vi "SSL Vision Log Player.vi"() -> ()   [LabVIEW 2016]
uses:
  SSL Referee Game Status.ctl
  GUI/IA Robot Line Display.ctl
  Filters/Estimadores.ctl
  SSL/SSL Field State.ctl
  SSL Detection Frame.ctl
  SSL Detection Robot.ctl
  SSL Detection Ball.ctl
  <extravilib>/ChannelInstances/Lossy Stream-t'SSL Field State.ctl'/Write With Abort.vi
  <extravilib>/ChannelInstances/Lossy Stream-t'SSL Referee Game Status.ctl'/Write With Abort.vi
  <extravilib>/ChannelInstances/Lossy Stream-t'SSL Referee Game Status.ctl'/Read With Abort.vi
  <extravilib>/ChannelInstances/Lossy Stream-t'SSL Field State.ctl'/Read With Abort.vi
  <extravilib>/ChannelInstances/Lossy Stream-t'AI Input.ctl'/Write With Abort.vi
  <extravilib>/ChannelInstances/Lossy Stream-t'AI Input.ctl'/Read With Abort.vi
  <extravilib>/ChannelInstances/Lossy Stream-t'SSL Field State.ctl'/Endpoint.vi
  <extravilib>/ChannelInstances/Lossy Stream-t'SSL Referee Game Status.ctl'/Endpoint.vi
  <extravilib>/ChannelInstances/Lossy Stream-t'AI Input.ctl'/Endpoint.vi
  <extravilib>/ChannelInstances/Lossy Stream-t'AI Input.ctl'/Instantiate.vi
  <extravilib>/ChannelInstances/Lossy Stream-t'AI Input.ctl'/)Channel.vi
  <resource>/ChannelSupport/_ChannelSupport/WaitIfNeeded.vi
  <extravilib>/ChannelInstances/Lossy Stream-t'SSL Referee Game Status.ctl'/Instantiate.vi
  <extravilib>/ChannelInstances/Lossy Stream-t'SSL Field State.ctl'/Instantiate.vi
  <extravilib>/ChannelInstances/Lossy Stream-t'SSL Referee Game Status.ctl'/)Channel.vi
  <extravilib>/ChannelInstances/Lossy Stream-t'SSL Field State.ctl'/)Channel.vi
  <extravilib>/ChannelInstances/Lossy Stream-a[.](u8)/Instantiate.vi
  <extravilib>/ChannelInstances/Stream-a[.](u8)/Instantiate.vi
  <extravilib>/ChannelInstances/Lossy Stream-t'SSL Referee Game Status.ctl'.lvlib
  <extravilib>/ChannelInstances/Lossy Stream-t'AI Input.ctl'.lvlib
  <extravilib>/ChannelInstances/Lossy Stream-t'SSL Field State.ctl'.lvlib
panel:
  in  "Estimador":T1
  out "Time Stamp":timestamp format="%<%.3X %x>T"
  out "error out 5":errorcluster
  out "error out 4":errorcluster
  out "Boolean":bool
  out "error out 3":errorcluster
  in  "Boolean 4":bool
  out "Boolean 3":bool
  in  "Port:":u16=10001
  in  "SSL Referee Address:":string="224.5.92.5"
  in  "Slide":i64(slide) min=0 max=47299339 scale=0.0..47299339.0
  out "offset (in bytes)":i64 format="%.3p"
  out "size (in bytes)":i64 format="%.3p"
  out "Boolean 2":bool
  in  "Modo":bool
  in  "Port:":u16=10020
  in  "file path (use dialog)":path=path "E:/Media/2016-07-01_cmdragons_immortals.log"
  in  "SSL Vision Address:":string="224.5.23.2"
  out "Role Playing FPS":dbl
  out "Total Delay":dbl format="%#.5g"
  in  "Goalie":string(combo)="Auto"
  in  "Command":string(combo)="Auto"
  in  "Time":enum16{"Azul", "Amarelo"}(ring) caption="Enum"
  in  "Lado":enum16{"Esquerdo", "Direito"}(ring) caption="Enum"
  in  "Role Decisor":enum16{"Simple Role Decisor", "No Role Decisor"}(ring)
  out "Game Status":T2={"Stage"="Normal First Half Pre", "Command"="Stop", "Time Left"=0.0, "Yellow Team"="", "Blue Team"="", "Yellow Score"=0, "Blue Score"=0, "Yellow Red Cards"=0, "Blue Red Cards"=0, "Yellow Yellow Cards"=0, "Blue Yellow Cards"=0, "Yellow Timeouts Left"=0, "Blue Timeouts Left"=0, "Yellow Timeout Remaining"=0.0, "Blue Timeout Remaining"=0.0, "Yellow Goalie Id"=0, "Blue Goalie Id"=0, "Time"=timestamp(2082758400 s since 1904-01-01)} {"Time" format="%<%.3X %x>T"; "Blue Timeout Remaining" format="%<%M:%S>t"; "Yellow Timeout Remaining" format="%<%M:%S>t"; "Time Left" format="%<%M:%S>t"}
  out "error out":errorcluster
  in  "Tab Control":enum32{"Robots", "Transmissão"}(tab)
  out "GUI Robot Array":T3[](array[typedef])
  in  "Serial TX":bool
  in  "UDP TX":bool=TRUE
  in  "Address:":string="127.0.0.1"
  in  "Port:":u16=20011
  in  "Porta:":refnum<visa-resource-name>
  out "Comm FPS":dbl
  out "error out 2":errorcluster
  # "UDP"
  # "LOG"
  # "Score"
  # "Red Cards"
  # "Yellow Cards"
  # "Timeouts Left"
  # "Timeout Remaining"
  # "Goalie ID"
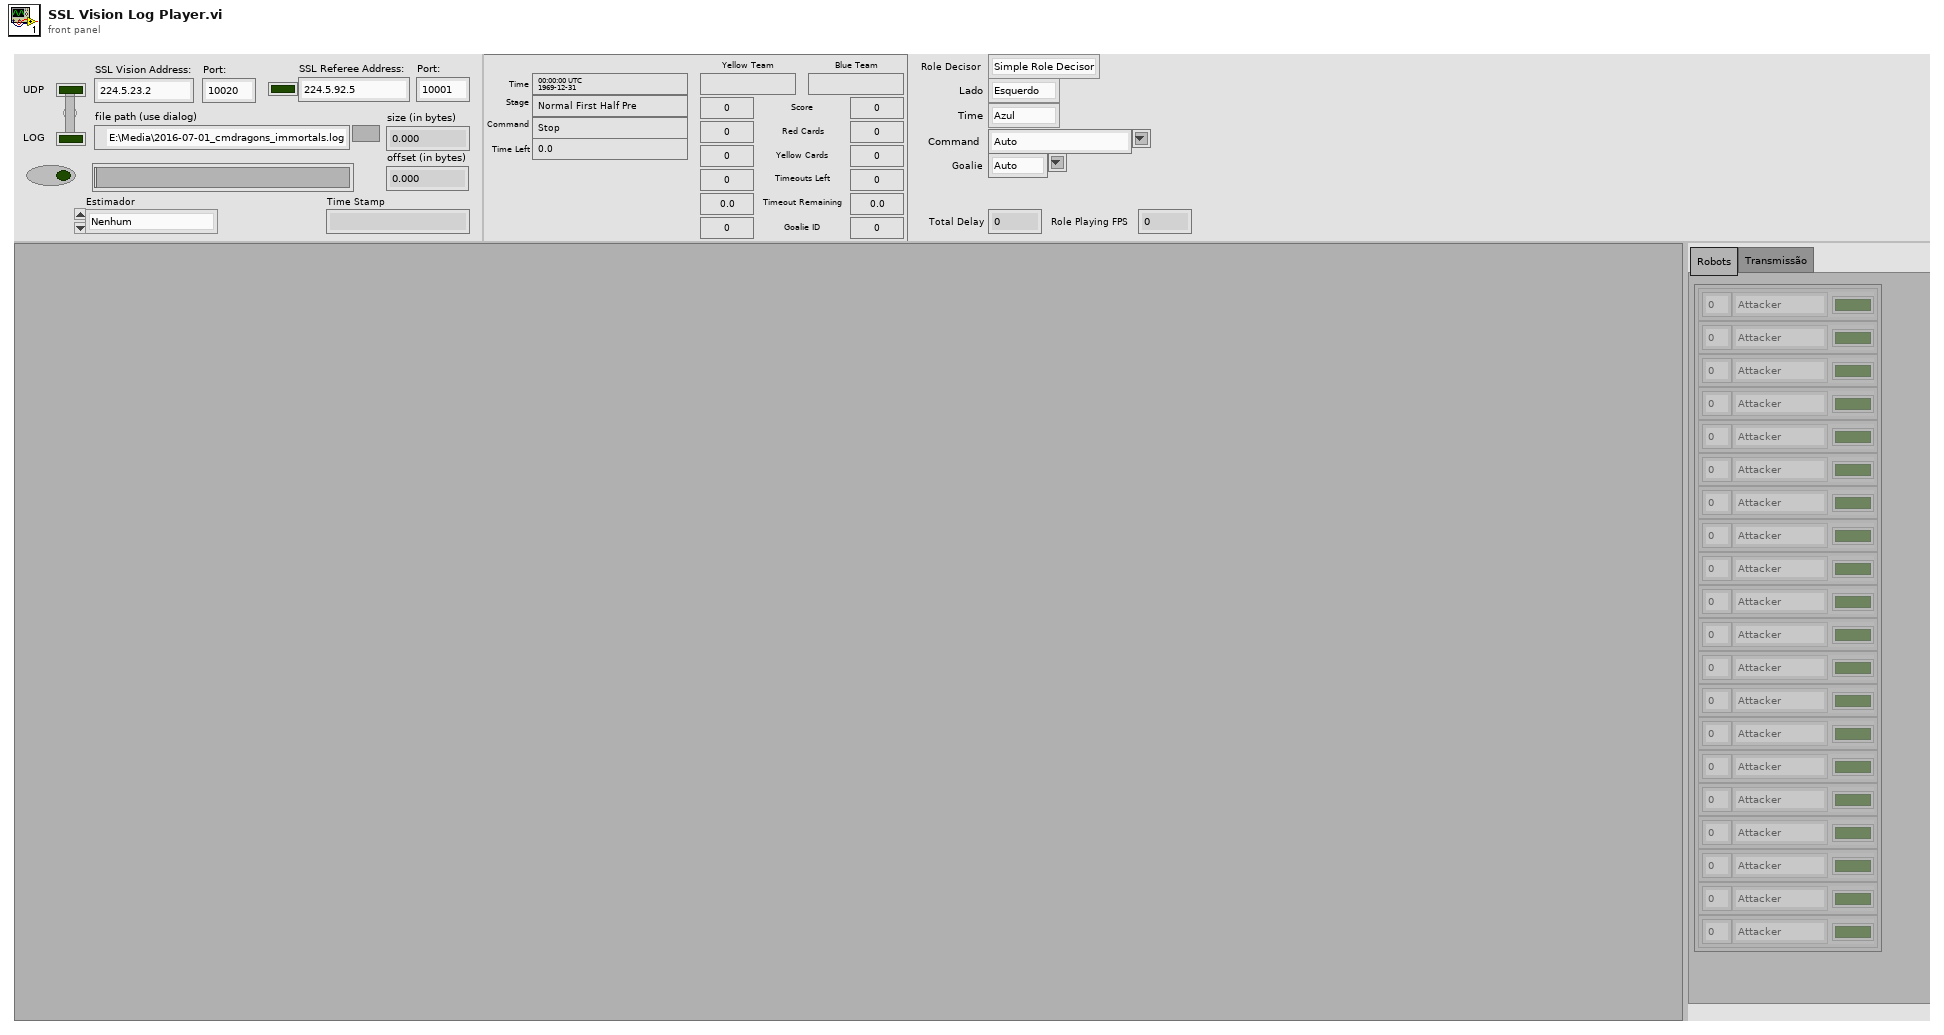
[diagram p1: front panel]
types:
  T1 = typedef "Estimadores.ctl" = enum16{"Nenhum", "Simples", "Simples Timestamp", "Simples Mult Cam", "Kalman", "Kalman Mult Cam"}
  T2 = typedef "SSL Referee Game Status.ctl" = cluster{"Stage":string, "Command":string, "Time Left":dbl, "Yellow Team":string, "Blue Team":string, "Yellow Score":u32, "Blue Score":u32, "Yellow Red Cards":u32, "Blue Red Cards":u32, "Yellow Yellow Cards":u32, "Blue Yellow Cards":u32, "Yellow Timeouts Left":u32, "Blue Timeouts Left":u32, "Yellow Timeout Remaining":dbl, "Blue Timeout Remaining":dbl, "Yellow Goalie Id":u32, "Blue Goalie Id":u32, "Time":timestamp}
  T3 = typedef "IA Robot Line Display.ctl" = cluster{"ID":dbl, "function":enum16{"Attacker", "Goalie", "Defender"}, "dribble":bool}
  T4 = typedef "Stream-a[.](u8).lvlib/)Channel.ctl" = refnum<queue>
  T5 = typedef "Lossy Stream-a[.](u8).lvlib/)Channel.ctl" = refnum<queue>
  T6 = typedef "SSL Field State.ctl" = cluster{"Detection Frame Out":T7, "Field Size Out":cluster{"line_width":u32, "field_length":u32, "field_width":u32, "boundary_width":u32, "referee_width":u32, "goal_width":u32, "goal_depth":u32, "goal_wall_width":u32, "center_circle_radius":u32, "defense_radius":u32, "defense_stretch":u32, "free_kick_from_defense_dist":u32, "penalty_spot_from_field_line_dist":u32, "penalty_line_from_spot_dist":u32}, "Received Time Stamp":timestamp}
  T7 = typedef "SSL Detection Frame.ctl" = cluster{"frame_number":u32, "t_capture":dbl, "t_sent":dbl, "camera_id":u32, "robots_yellow":T8[], "robots_blue":T8[], "balls":T9[], "Valid":bool, "Time Stamp":timestamp}
  T8 = typedef "SSL Detection Robot.ctl" = cluster{"x":sgl, "robot_id":u32, "confidence":sgl, "y":sgl, "orientation":sgl, "pixel_x":sgl, "pixel_y":sgl, "height":sgl, "Valid":bool, "Time Stamp":timestamp}
  T9 = typedef "SSL Detection Ball.ctl" = cluster{"x":sgl, "area":u32, "confidence":sgl, "y":sgl, "z":sgl, "pixel_x":sgl, "pixel_y":sgl, "Valid":bool, "Time Stamp":timestamp}
  T10 = cluster{"line_width":u32, "field_length":u32, "field_width":u32, "boundary_width":u32, "referee_width":u32, "goal_width":u32, "goal_depth":u32, "goal_wall_width":u32, "center_circle_radius":u32, "defense_radius":u32, "defense_stretch":u32, "free_kick_from_defense_dist":u32, "penalty_spot_from_field_line_dist":u32, "penalty_line_from_spot_dist":u32}
  T11 = typedef "Lossy Stream-t'SSL Field State.ctl'.lvlib/)Channel.ctl" = refnum<queue>
  T12 = typedef "SSL Referee.ctl" = cluster{"packet_\ntimestamp":u64, "stage":u64, "stage_time_left":i32, "command ":u64, "command_\ncounter ":u32, "command_\ntimestamp":u64, "yellow team info":T13, "blue team info":T13, "Point":cluster{"x":sgl, "y":sgl}}
  T13 = typedef "SSL Referee Team Info.ctl" = cluster{"name":string, "score":u32, "red_cards":u32, "yellow_cards_time":u32[], "yellow_cards":u32, "timeout":u32, "timeout_times":u32, "goalie":u32}
  T14 = typedef "Lossy Stream-t'SSL Referee Game Status.ctl'.lvlib/)Channel.ctl" = refnum<queue>
  T15 = typedef "AI Input.ctl" = cluster{"our_robots":T16[], "enemy_robots":T16[], "balls":T17[], "geometry":T18, "IA Judge":T19, "Received Timestamp":timestamp}
  T16 = typedef "AI Robot.ctl" = cluster{"id":u32, "function":enum16{"Attacker", "Goalie", "Defender"}, "x":dbl, "y":dbl, "orientation":dbl, "v_tangent":dbl, "v_normal":dbl, "v_ang":dbl, "kick_x":dbl, "kick_z":dbl, "dribble":bool, "Timestamp":timestamp, "dest_x":dbl, "dest_y":dbl, "dest_orientation":dbl}
  T17 = typedef "AI Ball.ctl" = cluster{"x":dbl, "y":dbl, "timestamp":timestamp}
  T18 = typedef "Field Size.ctl" = cluster{"line_width":u32, "field_length":u32, "field_width":u32, "boundary_width":u32, "referee_width":u32, "goal_width":u32, "goal_depth":u32, "goal_wall_width":u32, "center_circle_radius":u32, "defense_radius":u32, "defense_stretch":u32, "free_kick_from_defense_dist":u32, "penalty_spot_from_field_line_dist":u32, "penalty_line_from_spot_dist":u32}
  T19 = typedef "AI Judge.ctl" = cluster{"stage":string, "command":string, "our_goalie_id":dbl, "enemy_goalie_id":dbl, "command\nenum":T20, "Time":enum16{"Azul", "Amarelo"}}
  T20 = typedef "Command Enum.ctl" = enum16{"Halt", "Stop", "Force Start", "PKA Normal Start", "Prepare Kickoff Ally", "PKE Normal Start", "Prepare Kickoff Enemy", "Prepare Penalty Ally", "Prepare Penalty Enemy", "Direct Free Enemy", "Direct Free Ally", "Indirect Free Enemy", "Indirect Free Ally", "Timeout Enemy", "Timeout Ally", "Goal Enemy", "Goal Ally", "Ball Placement Enemy", "Ball Placement Ally", "None"}
  T21 = typedef "Lossy Stream-t'AI Input.ctl'.lvlib/)Channel.ctl" = refnum<queue>
  T22 = typedef "grSim Robot Command.ctl" = cluster{"id":u32, "kickspeedx":sgl, "kickspeedz":sgl, "veltangent":sgl, "velnormal":sgl, "velangular":sgl, "spinner":bool, "wheelspeed":bool, "wheel1":sgl, "wheel2":sgl, "wheel3":sgl, "wheel4":sgl}
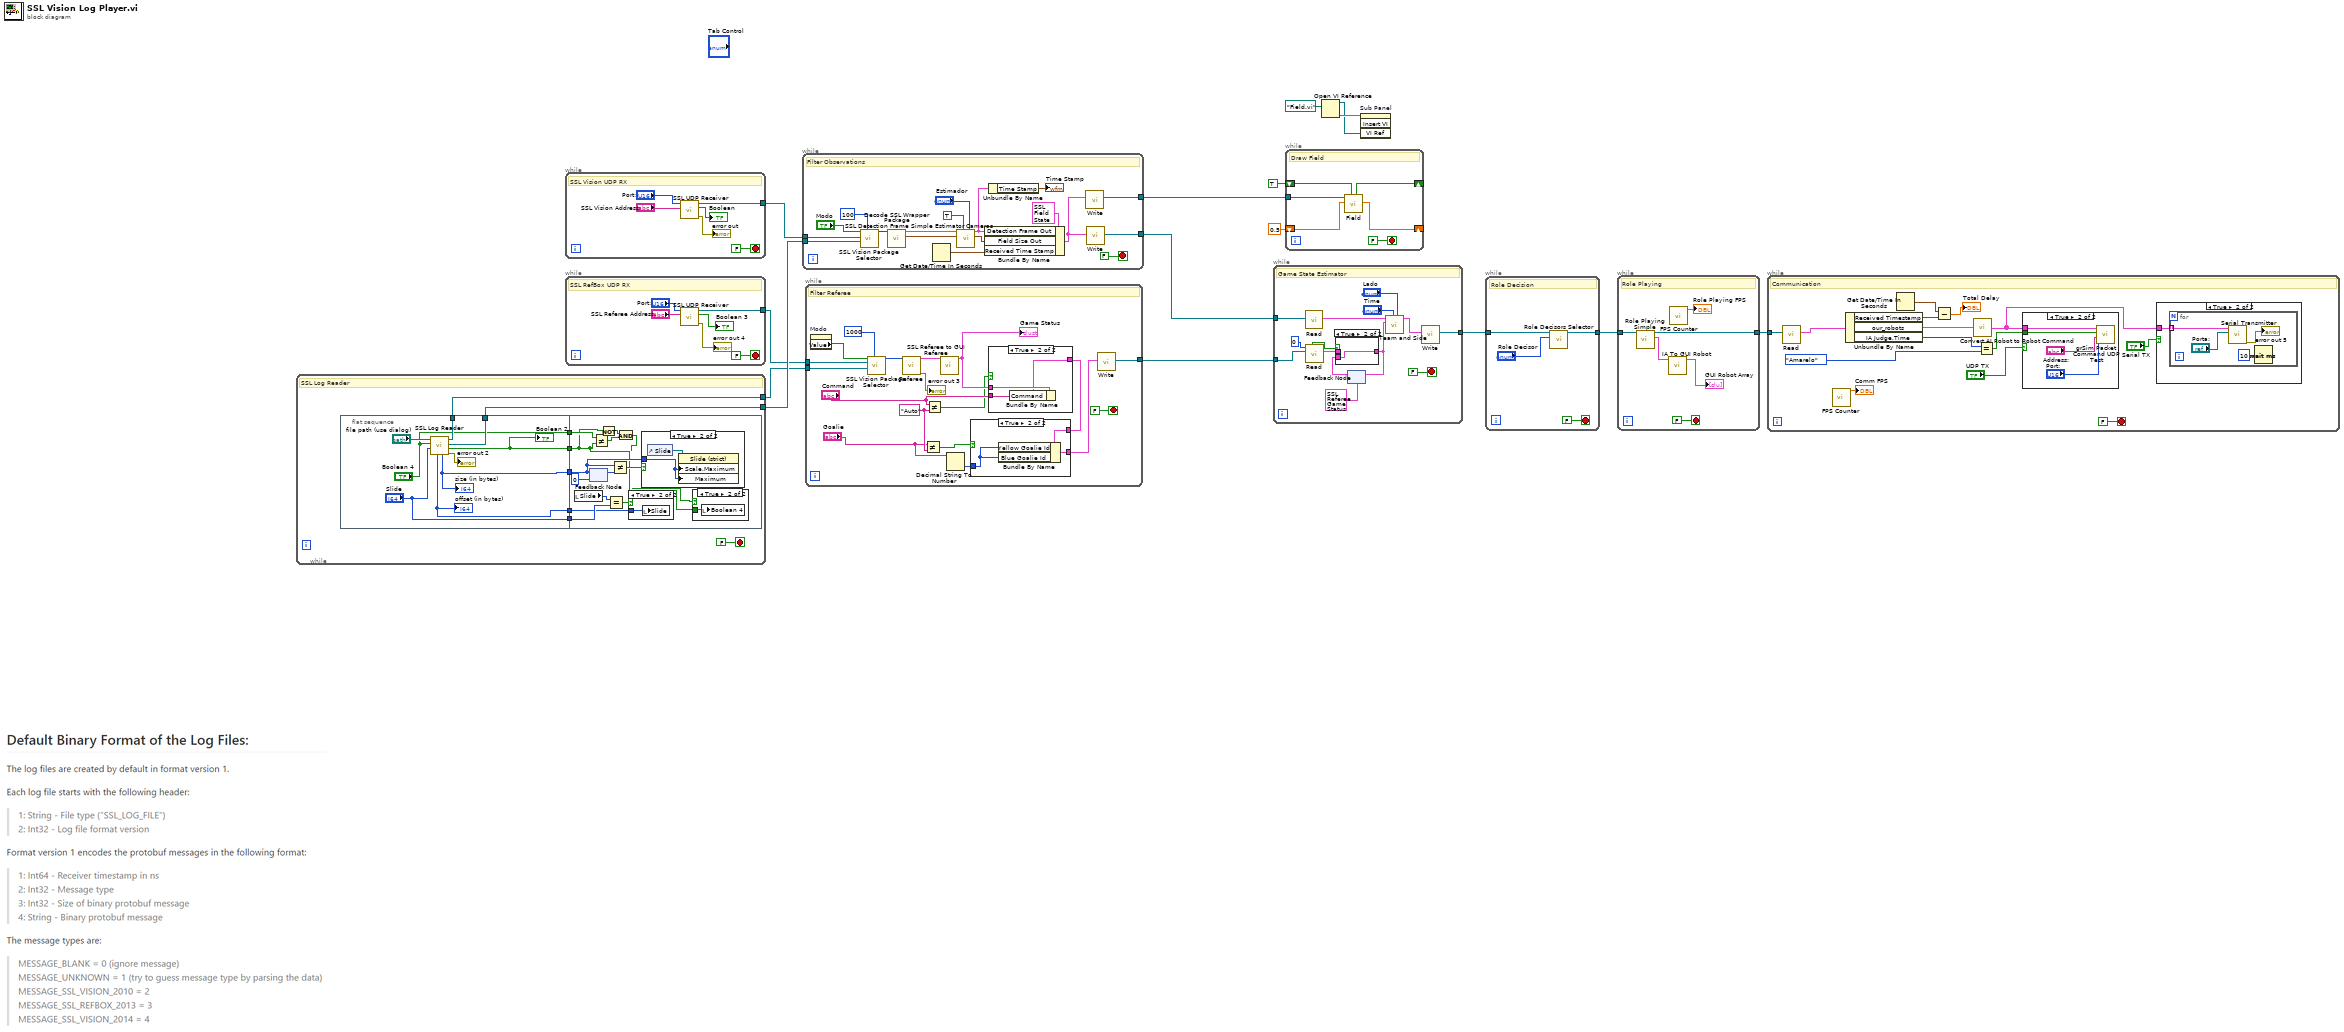
[diagram p0: block diagram]
diagram:
  n1 = while {
    tunnel: [w21] -> w15
    tunnel: [w22] -> w13
    stop <- FALSE stop-if-true
    # "SSL Log Reader"
    n2 = flat-sequence {
      tunnel: [w30] -> w22
      tunnel: [w29] -> w21
      tunnel: [w28] -> w20
      tunnel: ["Slide"] -> w19
      tunnel: [w26] -> w18
      tunnel: [w24] -> w17
      tunnel: ["Boolean 4"] -> w16
      tunnel: w20 -> [w42]
      tunnel: w19 -> [w44]
      tunnel: w18 -> [w39]
      tunnel: w17 -> [w35]
      tunnel: w16 -> [w37]
      frame #0 {
        n3 = call "SSL Log Reader.vi"("Slide"="Slide", "Boolean 4"="Boolean 4", "file path (use dialog)"="file path (use dialog)") -> ("error out"=→"error out 2":errorcluster, "Playing"=w24:bool, "channel 2"=w29:T4, "Channel out"=w30:T4, "size (in bytes)"=w26:i64, "offset (in bytes)"=w28:i64)  [unwired: 3 in]
        "size (in bytes)" <- w26
        "offset (in bytes)" <- w28
        "Boolean 2" <- w24
      }
      frame #1 {
        n4 = local read "Slide"() -> (w45:i64)
        n5 = feedback-in #1(w39) -> ()
        n6 = feedback #1(i64 0 ("size (in bytes)")) -> (w41:i64)
        n7 = Not Equal?(x=w37, y=w35) -> (x != y?=w36:bool)
        n8 = Not(x=w35) -> (.not. x?=w34:bool)
        n9 = Equal?(x=w45, y=w44) -> (x = y?=w43:bool)
        n10 = Not Equal?(x=w39, y=w41) -> (x != y?=w40:bool)
        n11 = And(x=w34, y=w36) -> (x .and. y?=w33:bool)
        n12 = case shown="True" w43 {
          tunnel: w42 -> [_ w49]
          frame False {
          }
          frame True {
            n13 = local write "Slide"(w49) -> ()
          }
        }
        n14 = case shown="True" w40 {
          tunnel: w39 -> [_ w47]
          frame False {
          }
          frame True {
            n15 = control-ref of="Slide"() -> (w48:refnum<vi>)
            n16 = property class="Slide (strict)"(reference=w48, "Scale.Maximum"=w47, "Maximum"=w47) -> ()  [unwired: 1 in, 2 out]
          }
        }
        n17 = case shown="True" w33 {
          tunnel: w35 -> [_ w46]
          frame False {
          }
          frame True {
            n18 = local write "Boolean 4"(w46) -> ()
          }
        }
      }
    }
  }
  n19 = while {
    tunnel: [w53] -> w14
    stop <- FALSE stop-if-true
    # "SSL Vision UDP RX"
    n20 = call "SSL UDP Receiver.vi"("SSL Vision Address:"="SSL Vision Address:", "Port:"="Port:") -> ("error out"=→"error out":errorcluster, "Boolean"=→"Boolean":bool, "Channel out"=w53:T5)  [unwired: 7 in]
  }
  n21 = while {
    tunnel: [w56] -> w6
    stop <- FALSE stop-if-true
    # "SSL RefBox UDP RX"
    n22 = call "SSL UDP Receiver.vi"("SSL Vision Address:"="SSL Referee Address:", "Port:"="Port:") -> ("error out"=→"error out 4":errorcluster, "Boolean"=→"Boolean 3":bool, "Channel out"=w56:T5)  [unwired: 7 in]
  }
  n23 = while {
    tunnel: w15 -> [w77]
    tunnel: w14 -> [w75]
    tunnel: [w67] -> w7
    tunnel: [w65] -> w5
    stop <- FALSE stop-if-true
    # "Filter Observations"
    n24 = call "SSL Vision Package Selector.vi"("timeout in ms (-1)"=100, "channel in"=w77, "Channel in"=w75, "Modo"="Modo") -> ("element"=w76:u8[])  [unwired: 7 in]
    n25 = call "Decode SSL Wrapper Package.vi"("unsigned byte array"=w76) -> ("Field Size"=w73:T10, "Detection Frame"=w78:T7)  [unwired: 7 in, 2 out]
    n26 = Get Date/Time In Seconds() -> (seconds since 1Jan1904=w69:timestamp)
    n27 = call "SSL Detection Frame Simple Estimator Cameras.vi"("Estimador"="Estimador", "Enable"=TRUE, "Field Size"=w73, "Detection Frame In"=w78) -> ("Field Size Out"=w68:T10, "Detection Frame Out"=w64:T7)  [unwired: 6 in]
    n28 = Bundle By Name(cluster=T6 {"Detection Frame Out"={"frame_number"=0, "t_capture"=0.0, "t_sent"=0.0, "camera_id"=0, "robots_yellow"=[], "robots_blue"=[], "balls"=[], "Valid"=FALSE, "Time Stamp"=timestamp(0 s since 1904-01-01)}, "Field Size Out"={"line_width"=0, "field_length"=0, "field_width"=0, "boundary_width"=0, "referee_width"=0, "goal_width"=0, "goal_depth"=0, "goal_wall_width"=0, "center_circle_radius"=0, "defense_radius"=0, "defense_stretch"=0, "free_kick_from_defense_dist"=0, "penalty_spot_from_field_line_dist"=0, "penalty_line_from_spot_dist"=0}, "Received Time Stamp"=timestamp(0 s since 1904-01-01)}, "Detection Frame Out"=w64, "Field Size Out"=w68, "Received Time Stamp"=w69) -> (w66:T6)
    n29 = Unbundle By Name(w64) -> ("Time Stamp"=→"Time Stamp":timestamp)
    n30 = call <extravilib>:"Write.vi"("element"=w66) -> ("channel"=w67:T11)  [unwired: 8 in, 2 out]
    n31 = call <extravilib>:"Write.vi"("element"=w66) -> ("channel"=w65:T11)  [unwired: 8 in, 2 out]
  }
  n32 = while {
    tunnel: w13 -> [w91]
    tunnel: w6 -> [w92]
    tunnel: [w89] -> w4
    stop <- FALSE stop-if-true
    w85 = "Auto" ("y")
    # "Filter Referee"
    n33 = property on="Modo" class="Bool (strict)"() -> ("Value"=w93:bool)  [unwired: 2 in, 2 out]
    n34 = call "SSL Vision Package Selector.vi"("timeout in ms (-1)"=1000, "channel in"=w91, "Channel in"=w92, "Modo"=w93) -> ("element"=w94:u8[])  [unwired: 7 in]
    n35 = call "Referee.vi"("element"=w94) -> ("output cluster"=w95:T12, "error out"=→"error out 3":errorcluster)  [unwired: 13 in]
    n36 = Not Equal?(x="Goalie", y=w85) -> (x != y?=w84:bool)
    n37 = Not Equal?(x="Command", y=w85) -> (x != y?=w86:bool)
    n38 = call "SSL Referee to GUI Referee.vi"("SSL Game Status"=w95) -> ("GUI Game Status"=w88:T2)  [unwired: 10 in]
    "Game Status" <- w88
    n39 = Decimal String To Number(string="Goalie") -> (number=w80:i32)  [unwired: 2 in, 1 out]
    n40 = case shown="True" w86 {
      tunnel: w88 -> [w102 w105]
      tunnel: [w102 w104] -> w83
      tunnel: "Command" -> [_ w103]
      frame False {
      }
      frame True {
        n41 = Bundle By Name(cluster=w105, "Command"=w103) -> (w104:T2)
      }
    }
    n42 = case shown="True" w84 {
      tunnel: w83 -> [w98 w101]
      tunnel: [w98 w100] -> w82
      tunnel: w80 -> [_ w99]
      frame False {
      }
      frame True {
        n43 = Bundle By Name(cluster=w101, "Yellow Goalie Id"=w99, "Blue Goalie Id"=w99) -> (w100:T2)
      }
    }
    n44 = call <extravilib>:"Write.vi"("element"=w82) -> ("channel"=w89:T14)  [unwired: 8 in, 2 out]
  }
  n45 = while {
    tunnel: w5 -> [w107]
    tunnel: w4 -> [w118]
    tunnel: [w111] -> w3
    stop <- FALSE stop-if-true
    # "Game State Estimator"
    n46 = call <extravilib>:"Read.vi"("channel"=w107) -> ("element"=w106:T6)  [unwired: 5 in, 5 out]
    n47 = call <extravilib>:"Read.vi"("channel"=w118, "timeout in ms (-1)"=0) -> ("element"=w115:T2, "timed out?"=w116:bool)  [unwired: 4 in, 4 out]
    n48 = feedback #2(T2 {"Stage"="First Half", "Command"="Stop", "Time Left"=0.0, "Yellow Team"="", "Blue Team"="", "Yellow Score"=0, "Blue Score"=0, "Yellow Red Cards"=0, "Blue Red Cards"=0, "Yellow Yellow Cards"=0, "Blue Yellow Cards"=0, "Yellow Timeouts Left"=0, "Blue Timeouts Left"=0, "Yellow Timeout Remaining"=0.0, "Blue Timeout Remaining"=0.0, "Yellow Goalie Id"=0, "Blue Goalie Id"=0, "Time"=timestamp(0 s since 1904-01-01)} ("element")) -> (w114:T2)
    n49 = case shown="True" w116 {
      tunnel: w115 -> [w120 _]
      tunnel: [w120 w121] -> w113
      tunnel: w114 -> [_ w121]
      frame False {
      }
      frame True {
      }
    }
    n50 = feedback-in #2(w113) -> ()
    n51 = call "Team and Side.vi"("Lado"="Lado", "Time"="Time", "Game Status"=w113, "Field State Input"=w106) -> ("IA State"=w112:T15)  [unwired: 7 in]
    n52 = call <extravilib>:"Write.vi"("element"=w112) -> ("channel"=w111:T21)  [unwired: 8 in, 2 out]
  }
  n53 = while {
    shift-right: [w125] -> _
    shift-left: 0.5 ("New Scale") -> [w127]
    shift-right: [w124] -> _
    shift-left: TRUE ("AutoScale Out") -> [w123]
    tunnel: w7 -> [w122]
    stop <- FALSE stop-if-true
    # "Draw Field"
    n54 = call "Field.vi"("AutoScale"=w123, "Scale mm/pixel"=w127, "channel"=w122) -> ("Scale Out"=w125:dbl, "AutoScale Out"=w124:bool)  [unwired: 6 in, 1 out]
  }
  n55 = Open VI Reference(vi path=path "Field.vi") -> (vi reference=w10:refnum<vi>, error out=w11:errorcluster)  [unwired: 5 in]
  n56 = invoke on="Sub Panel" class="SubPnl" method="Insert VI"(error in=w11, "VI Ref"=w10) -> ()  [unwired: 2 in, 4 out]
  n57 = while {
    tunnel: w3 -> [w128]
    tunnel: [w130] -> w2
    stop <- FALSE stop-if-true
    # "Role Decision"
    n58 = call "Role Decisors Selector.vi"("Role Decisor"="Role Decisor", "channel"=w128) -> ("channel 2"=w130:T21)  [unwired: 8 in, 1 out]
  }
  n59 = while {
    tunnel: w2 -> [w136]
    tunnel: [w135] -> w1
    stop <- FALSE stop-if-true
    # "Role Playing"
    n60 = call "Role Playing Simple.vi"("channel"=w136) -> ("IA State Output"=w134:T15, "channel 2"=w135:T21)  [unwired: 9 in]
    n61 = call "IA To GUI Robot.vi"("Output IA"=w134) -> ("GUI Robot Array"=→"GUI Robot Array":T3[])  [unwired: 10 in]
    n62 = call "FPS Counter.vi"() -> ("Numeric"=→"Role Playing FPS":dbl)  [unwired: 11 in]
  }
  n63 = while {
    tunnel: w1 -> [w150]
    stop <- FALSE stop-if-true
    # "Communication"
    n64 = call <extravilib>:"Read.vi"("channel"=w150) -> ("element"=w149:T15)  [unwired: 5 in, 5 out]
    n65 = call "FPS Counter.vi"() -> ("Numeric"=→"Comm FPS":dbl)  [unwired: 11 in]
    n66 = Unbundle By Name(w149) -> ("Received Timestamp"=w144:timestamp, "our_robots"=w148:T16[], "IA Judge.Time"=w147:enum16{"Azul", "Amarelo"})
    n67 = Get Date/Time In Seconds() -> (seconds since 1Jan1904=w143:timestamp)
    n68 = Subtract(x=w143, y=w144) -> (x-y=→"Total Delay":dbl)
    n69 = call "Convert AI Robot to Robot Command.vi"("Input Array"=w148) -> ("Output Array"=w141:T22[])
    n70 = Equal?(x=w147, y=enum16{"Azul", "Amarelo"}."Amarelo") -> (x = y?=w145:bool)
    n71 = case shown="True" "UDP TX" {
      tunnel: w145 -> [_ w160]
      tunnel: w141 -> [_ w157]
      frame False {
      }
      frame True {
        n72 = call "grSim Packet Command UDP Test.vi"("Port:"="Port:", "SSL Vision Address:"="Address:", "isteamyellow"=w160, "Robots"=w157) -> ()  [unwired: 8 in]
      }
    }
    n73 = case shown="True" "Serial TX" {
      tunnel: w141 -> [_ w152]
      frame False {
      }
      frame True {
        n74 = for {
          tunnel: w152 -> [w156] mode=indexing
          n75 = call "Serial Transmitter.vi"("Porta:"="Porta:", "Robots"=w156) -> ("error out"=→"error out 5":errorcluster)  [unwired: 9 in]
          n76 = Wait (ms)(milliseconds to wait=u32 10) -> ()  [unwired: 1 out]
        }
      }
    }
  }
